vi "API Set Stop.vi"(8 "error in":errorcluster, 11 "VISA resource name":refnum<visa-resource-name>) -> (0 "error out":errorcluster, 3 "VISA resource name out":refnum<visa-resource-name>)   [LabVIEW 2024, in "Thermotron 8800.lvlib"]
uses:
  Thermotron 8800.lvlib
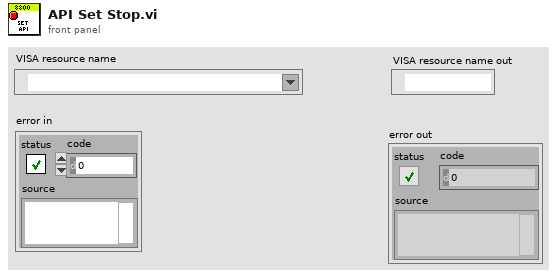
[diagram p1: front panel]
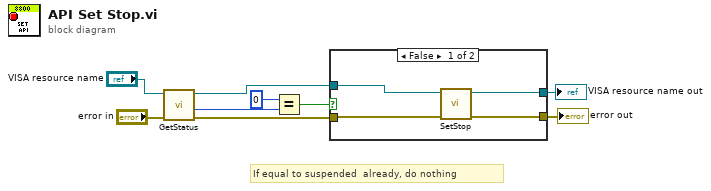
[diagram p0: block diagram]
diagram:
  # "If equal to suspended  already, do nothing"
  n1 = call "GetStatus.vi"("error in"="error in", "VISA resource name"="VISA resource name") -> ("error out"=w5:errorcluster, "Status word"=w6:i32, "VISA resource name out"=w7:refnum<visa-resource-name>)  [unwired: 6 in, 1 out]
  n2 = Equal?(x=0, y=w6) -> (x = y?=w8:bool)
  n3 = case shown="False" w8 {
    tunnel: [w12 w15] -> w3
    tunnel: [w10 w14] -> w2
    tunnel: w5 -> [w11 w14]
    tunnel: w7 -> [w13 w15]
    frame False {
      n4 = call "SetStop.vi"("error in"=w11, "VISA resource name"=w13) -> ("error out"=w10:errorcluster, "VISA resource name out"=w12:refnum<visa-resource-name>)  [unwired: 8 in]
    }
    frame True {
    }
  }
  "VISA resource name out" <- w3
  "error out" <- w2
